vi "Create NI 9475 - PWM Output.vi"(8 "error in":errorcluster, 11 "channel settings":T1[](array[typedef])) -> (0 "error out":errorcluster, 3 "NI 9475 out":refnum<class "NI 9475.lvclass">)   [LabVIEW 2017, in "Scan Engine Scripting.lvlib" / "NI 9475.lvclass"]
uses:
  NI 9475.lvclass
  C:/Users/nitest/Documents/niveristand-scan-engine-ethercat-custom-device/Custom Device Source/Scripting/Modules/Module/Module.lvclass
  Channel Classes/PWM Output Channel/Frequency.ctl
  Channel Classes/PWM Output Channel/PWM Output Channel.lvclass
  Mode Classes/Controls/pwm channel settings.ctl
  Scan Engine Scripting.lvlib
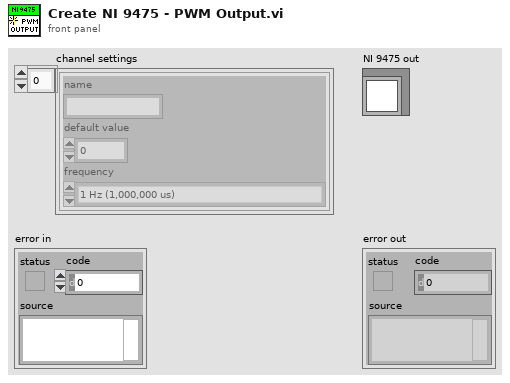
[diagram p1: front panel]
types:
  T1 = typedef "Scan Engine Scripting.lvlib/pwm channel settings.ctl" = cluster{"name":string, "default value":dbl, "frequency":T2}
  T2 = typedef "Scan Engine Scripting.lvlib/PWM Output Channel.lvclass/Frequency.ctl" = enum16{"1 Hz (1,000,000 us)", "50 Hz (20,000 us)", "250 Hz (4,000 us)", "500 Hz (2,000 us)", "1 kHz (1,000 us)", "5 kHz (200 us)", "10 kHz (100 us)", "20 kHz (50 us)"}
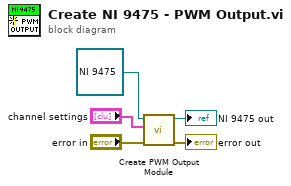
[diagram p0: block diagram]
diagram:
  n1 = call "Create PWM Output Module.vi"("error in (no error)"="error in", "channel settings"="channel settings", "module in"=refnum<class "NI 9475.lvclass"> refnum ("NI 9475 in")) -> ("error out"=→"error out":errorcluster, "module out"=→"NI 9475 out":refnum<class "NI 9475.lvclass">)  [unwired: 7 in]
